vi "SwerveAngleChooser.vi"(8 "Goal Override":bool, 9 "Hysteresis (deg)":dbl=10.0 format="%#_13g", 10 "Goal Angle (deg) [-180,+180]":dbl format="%#_13g", 11 "Current Angle (deg) [-180,+180]":dbl format="%#_13g") -> (2 "Flip Drive Motor Direction":bool, 3 "Angular Distance (deg)":dbl format="%_4g")   [LabVIEW 2020]
panel:
  in  "Goal Override Angle (deg) [-180,+180]":dbl format="%#_13g"
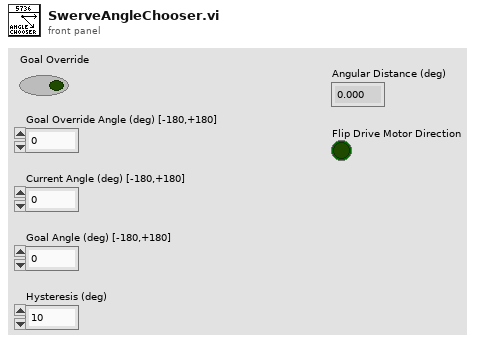
[diagram p1: front panel]
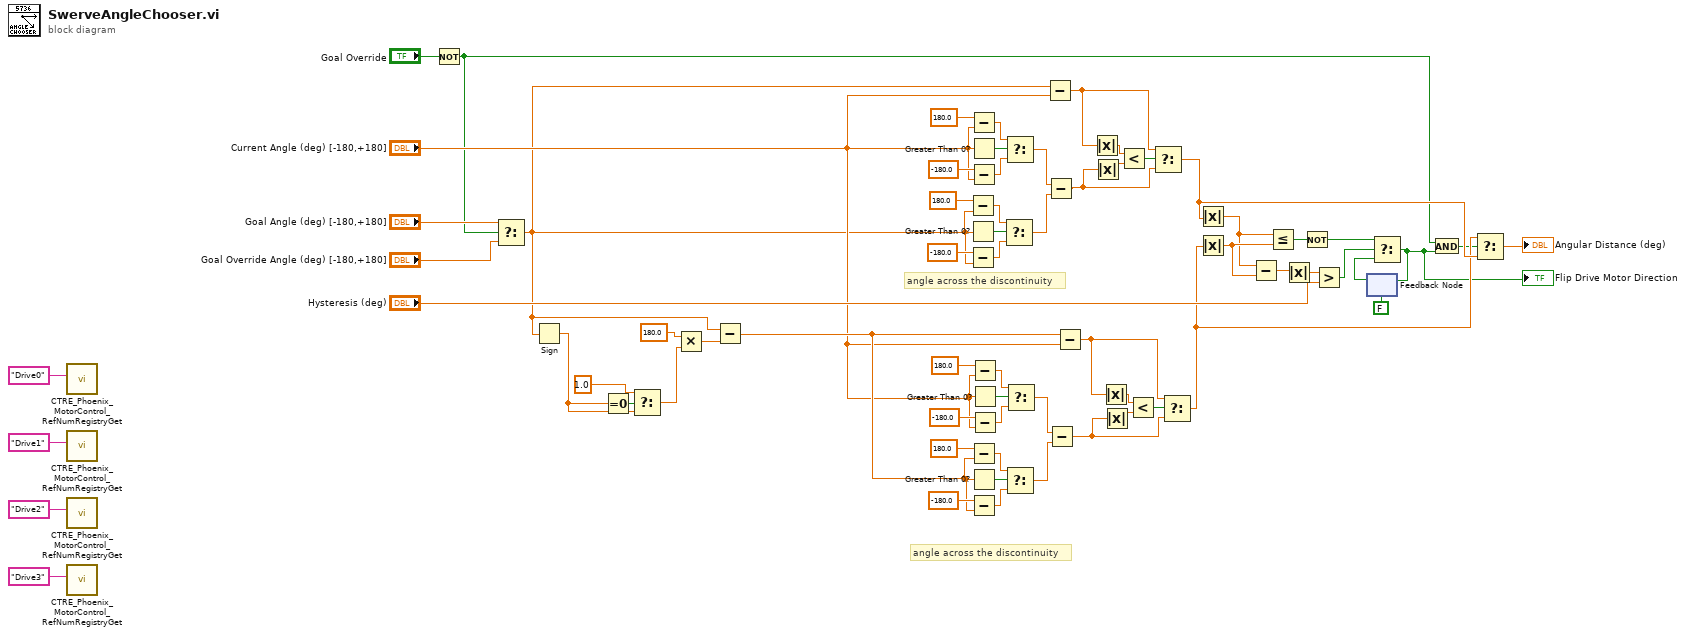
[diagram p0: block diagram]
diagram:
  # "angle across the discontinuity"
  # "angle across the discontinuity"
  n1 = call <vilib>:"CTRE_Phoenix_MotorControl_RefNumRegistryGet.vi"("refnum name"="Drive0") -> ()  [unwired: 9 in, 2 out]
  n2 = call <vilib>:"CTRE_Phoenix_MotorControl_RefNumRegistryGet.vi"("refnum name"="Drive1") -> ()  [unwired: 9 in, 2 out]
  n3 = call <vilib>:"CTRE_Phoenix_MotorControl_RefNumRegistryGet.vi"("refnum name"="Drive2") -> ()  [unwired: 9 in, 2 out]
  n4 = call <vilib>:"CTRE_Phoenix_MotorControl_RefNumRegistryGet.vi"("refnum name"="Drive3") -> ()  [unwired: 9 in, 2 out]
  n5 = Not(x="Goal Override") -> (.not. x?=w5:bool)
  n6 = Select(t="Goal Angle (deg) [-180,+180]", s=w5, f="Goal Override Angle (deg) [-180,+180]") -> (s? t:f=w9:dbl)
  n7 = Sign(1:w9) -> (0:w17:dbl)
  n8 = Equal To 0?(x=w17) -> (x = 0?=w18:bool)
  n9 = Select(t=1.0, s=w18, f=w17) -> (s? t:f=w14:dbl)
  n10 = Multiply(x=180.0 ("y"), y=w14) -> (x*y=w66:dbl)
  n11 = Subtract(x=w9, y=w66) -> (x-y=w39:dbl)
  n12 = Subtract(x=180.0, y=w9) -> (x-y=w27:dbl)
  n13 = Greater Than 0?(x=w9) -> (x > 0?=w29:bool)
  n14 = Subtract(x=-180.0, y=w9) -> (x-y=w25:dbl)
  n15 = Subtract(x=180.0, y="Current Angle (deg) [-180,+180]") -> (x-y=w32:dbl)
  n16 = Greater Than 0?(x="Current Angle (deg) [-180,+180]") -> (x > 0?=w34:bool)
  n17 = Subtract(x=-180.0, y="Current Angle (deg) [-180,+180]") -> (x-y=w30:dbl)
  n18 = Subtract(x=180.0, y=w39) -> (x-y=w48:dbl)
  n19 = Greater Than 0?(x=w39) -> (x > 0?=w50:bool)
  n20 = Subtract(x=-180.0, y=w39) -> (x-y=w46:dbl)
  n21 = Subtract(x=180.0, y="Current Angle (deg) [-180,+180]") -> (x-y=w54:dbl)
  n22 = Greater Than 0?(x="Current Angle (deg) [-180,+180]") -> (x > 0?=w56:bool)
  n23 = Subtract(x=-180.0, y="Current Angle (deg) [-180,+180]") -> (x-y=w52:dbl)
  n24 = Select(t=w27, s=w29, f=w25) -> (s? t:f=w23:dbl)
  n25 = Select(t=w32, s=w34, f=w30) -> (s? t:f=w24:dbl)
  n26 = Select(t=w48, s=w50, f=w46) -> (s? t:f=w44:dbl)
  n27 = Select(t=w54, s=w56, f=w52) -> (s? t:f=w45:dbl)
  n28 = Subtract(x=w9, y="Current Angle (deg) [-180,+180]") -> (x-y=w35:dbl)
  n29 = Subtract(x=w24, y=w23) -> (x-y=w21:dbl)
  n30 = Subtract(x=w45, y=w44) -> (x-y=w43:dbl)
  n31 = Subtract(x=w39, y="Current Angle (deg) [-180,+180]") -> (x-y=w40:dbl)
  n32 = Absolute Value(x=w35) -> (abs(x)=w36:dbl)
  n33 = Absolute Value(x=w21) -> (abs(x)=w37:dbl)
  n34 = Absolute Value(x=w40) -> (abs(x)=w41:dbl)
  n35 = Absolute Value(x=w43) -> (abs(x)=w42:dbl)
  n36 = Less?(x=w36, y=w37) -> (x < y?=w38:bool)
  n37 = Less?(x=w41, y=w42) -> (x < y?=w51:bool)
  n38 = Select(t=w35, s=w38, f=w21) -> (s? t:f=w13:dbl)
  n39 = Select(t=w40, s=w51, f=w43) -> (s? t:f=w12:dbl)
  n40 = Absolute Value(x=w13) -> (abs(x)=w57:dbl)
  n41 = Absolute Value(x=w12) -> (abs(x)=w58:dbl)
  n42 = Subtract(x=w57, y=w58) -> (x-y=w62:dbl)
  n43 = Less Or Equal?(x=w57, y=w58) -> (x <= y?=w20:bool)
  n44 = Absolute Value(x=w62) -> (abs(x)=w61:dbl)
  n45 = Not(x=w20) -> (.not. x?=w19:bool)
  n46 = Greater?(x=w61, y="Hysteresis (deg)") -> (0:w59:bool)
  n47 = feedback #1(FALSE) -> (w64:bool)
  n48 = Select(t=w19, s=w59, f=w64) -> (s? t:f=w10:bool)
  "Flip Drive Motor Direction" <- w10
  n49 = feedback-in #1(w10) -> ()
  n50 = And(x=w5, y=w10) -> (x .and. y?=w11:bool)
  n51 = Select(t=w12, s=w11, f=w13) -> (s? t:f=→"Angular Distance (deg)":dbl)
